vi "test-CSM mode.vi"(8 "error in (no error)":errorcluster, 11 "TestCase in":refnum<class "testcase-CSMAttributes.lvclass">) -> (0 "error out":errorcluster, 3 "TestCase out":refnum<class "testcase-CSMAttributes.lvclass">)   [LabVIEW 2017, in "testcase-CSMAttributes.lvclass"]
uses:
  testcase-CSMAttributes.lvclass
  5e1fa0b9-9953-4aea-b14f-852d0926f464.vi
  ca6da20f-918c-4697-94f5-fe779df5fb56.vi
  b6cafa74-5be5-493d-85c2-392da22f0834.vi
  474ebc5b-ede4-4fe2-a33b-3b2c34e901f1.vi
  6dc37769-ead1-45fc-a673-d21298543349.vi
  2b38d03e-680a-4e35-9447-0bd23ed7c194.vi
  aa53e100-d513-4525-b5da-2cac676b671d.vi
  src/user.lib/_NEVSTOP/Communicable State Machine(CSM)/AdvanceAPI/CSM - Set Module Attribute.vi
  src/user.lib/_NEVSTOP/Communicable State Machine(CSM)/AdvanceAPI/CSM - Get Module Attribute.vi
  <vilib>/addons/_JKI Toolkits/VI Tester/TestCase.llb/TestCase.lvclass
  src/user.lib/_NEVSTOP/Communicable State Machine(CSM)/Communicable State Machine.lvlib
  C:/Program Files (x86)/National Instruments/LabVIEW 2017/vi.lib/addons/_JKI Toolkits/VI Tester/TestCase.llb/TestCase.lvclass
panel:
  out "error out":errorcluster
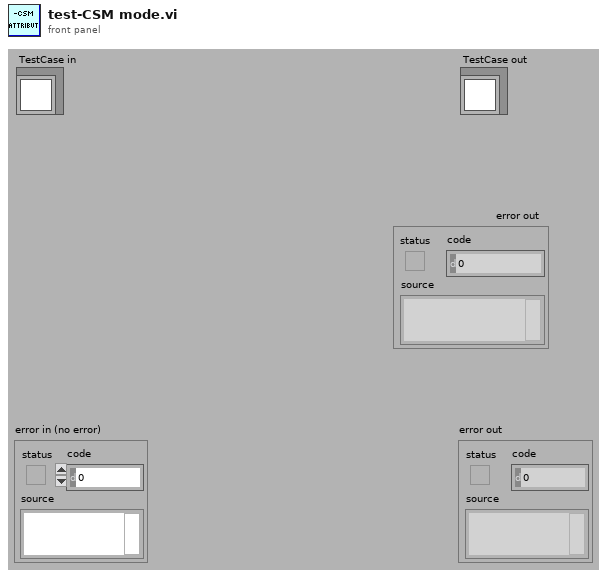
[diagram p1: front panel]
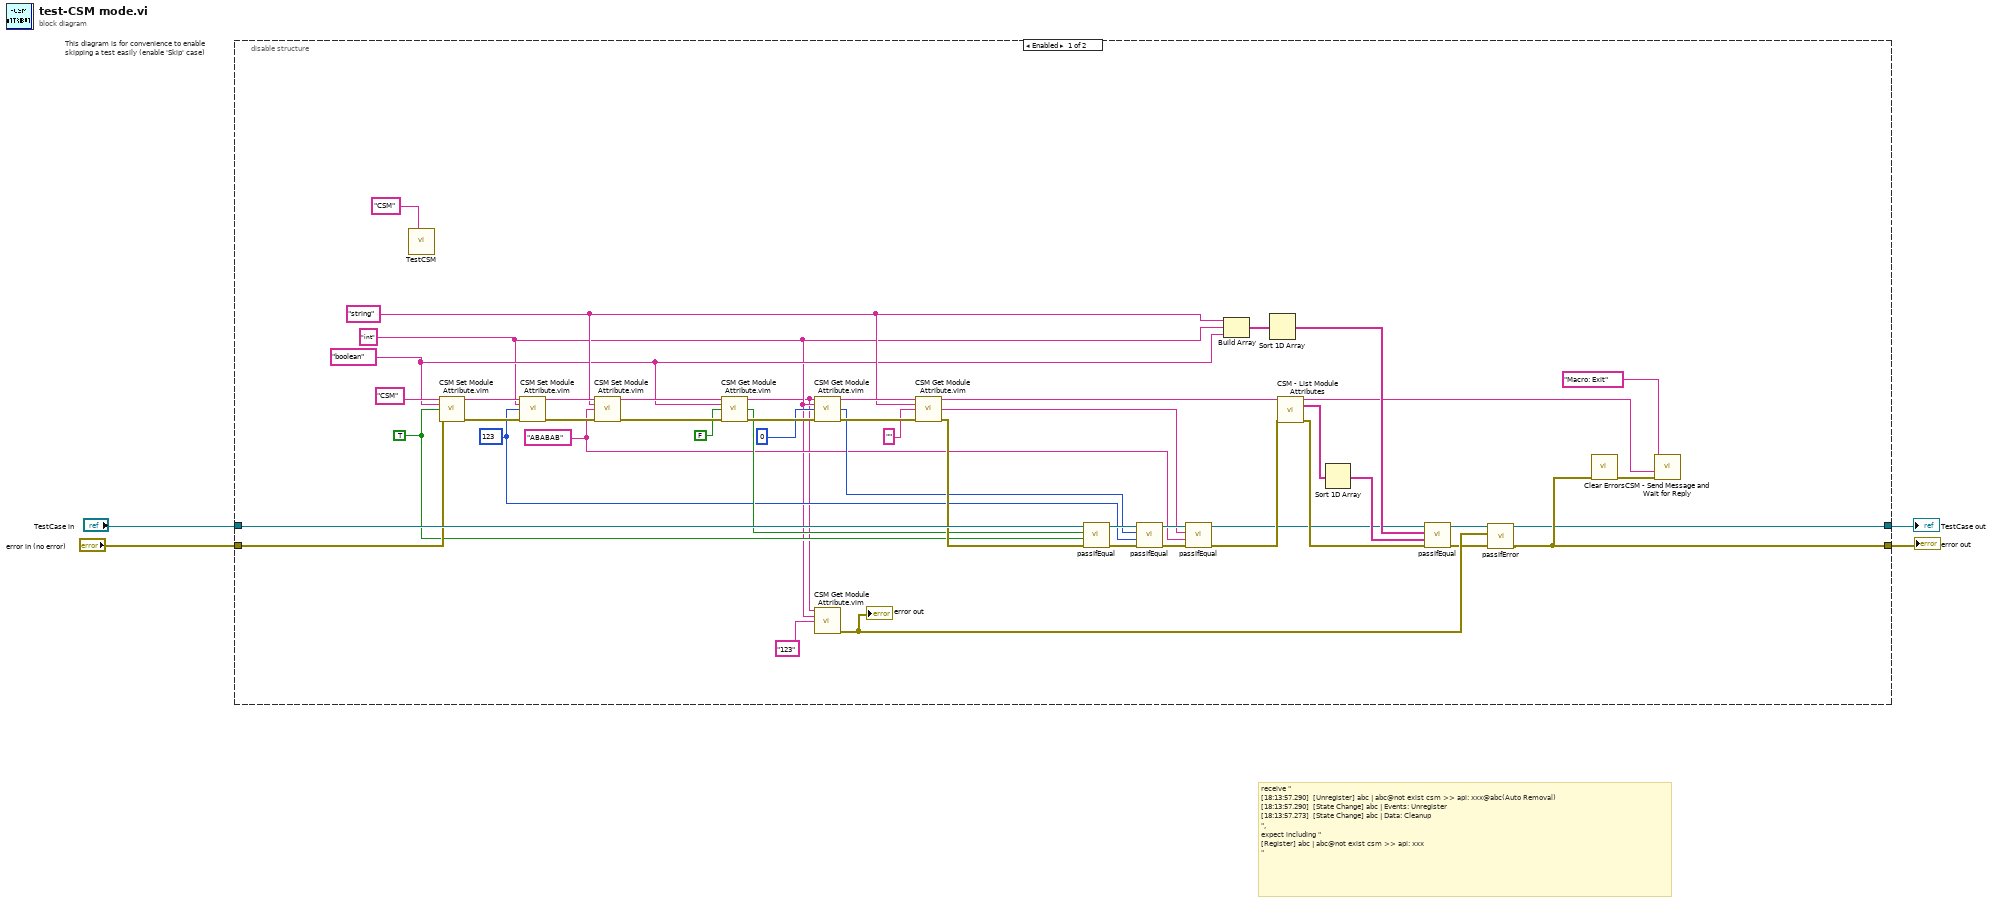
[diagram p0: block diagram]
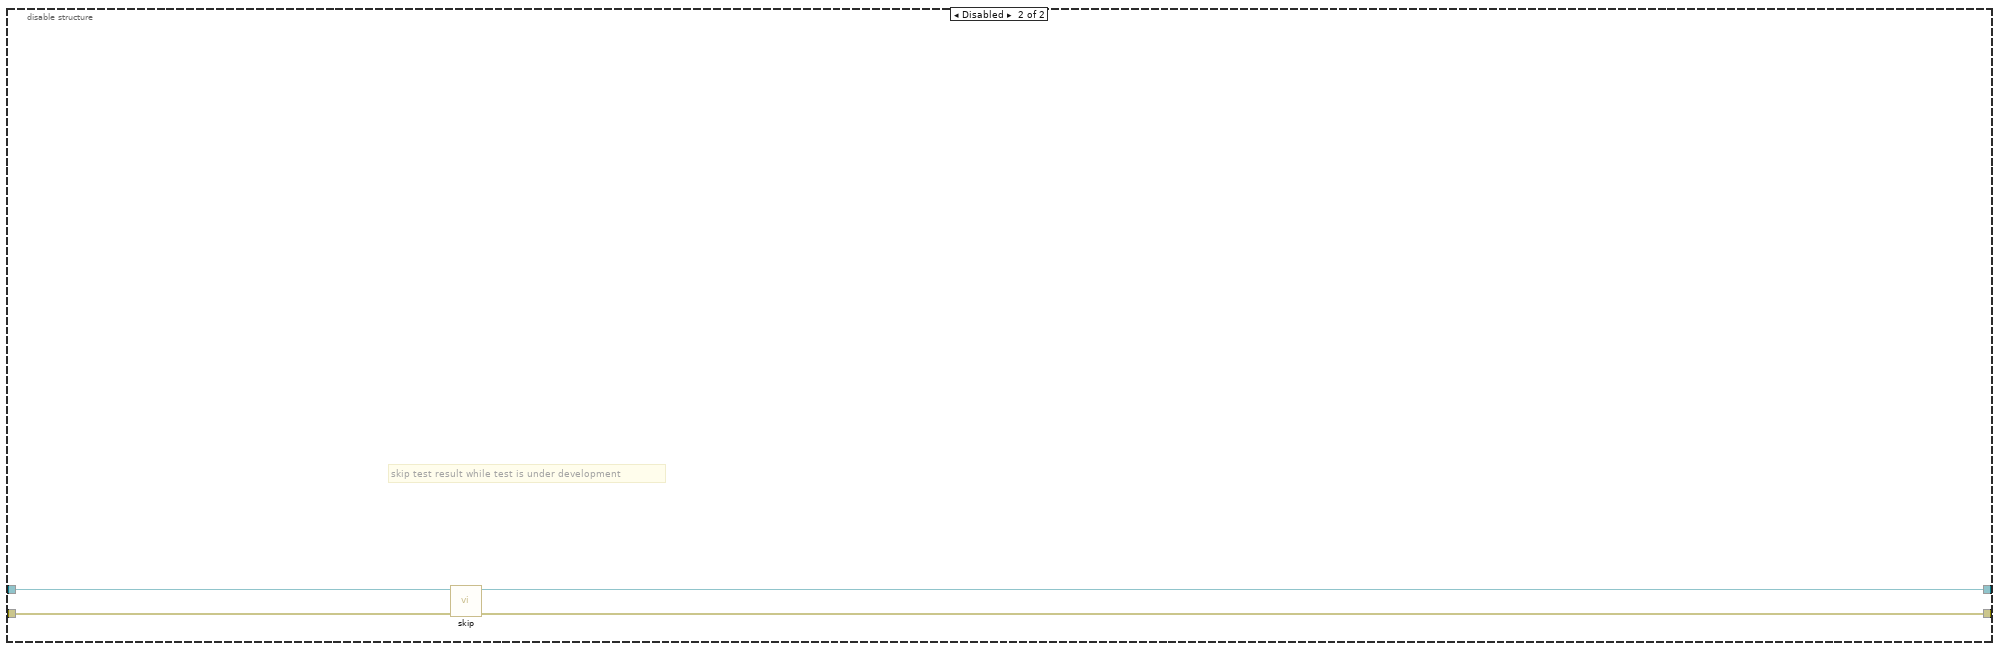
[diagram p2: hidden frame]
diagram:
  # "receive \"\n[18:13:57.290]  [Unregister] abc | abc@not exist csm >> api: xxx@abc(Auto Removal)\n[18:13:57.290]  [State Change] abc | Events: Unregister\n[18:13:57.273]  [State Change] abc | Data: Cleanup\n\", \nexpect including \"\n[Register] abc | abc@not exist csm >> api: xxx\n\""
  n1 = disable-structure "This diagram is for convenience to enable skipping a test easily (enable 'Skip' case)" shown="Enabled" {
    disable-tunnel: "TestCase in" -> [w52 w56]
    disable-tunnel: [w5 w54] -> w1
    disable-tunnel: [w6 w55] -> w3
    disable-tunnel: "error in (no error)" -> [w51 w53]
    frame Enabled {
      w26 = "ABABAB" ("Attribute")
      w22 = "string" ("Attribute")
      w30 = 123
      w11 = "int" ("Attribute")
      w35 = TRUE
      w21 = "boolean" ("Attribute")
      n2 = call "TestCSM.vi"("Name (\"\" to Use UUID)"="CSM" ("Name (\"\" to Use UUID)")) -> ()  [unwired: 11 in]
      n3 = call "CSM Set Module Attribute.vim"("CSM Name"="CSM" ("Name (\"\" to Use UUID)"), "Attribute"=w21, "Value"=w35, "Error In"=w51) -> ("CSM Name (Dup)"=w46:string, "error out"=w48:errorcluster)  [unwired: 8 in, 2 out]
      n4 = call "CSM Set Module Attribute.vim"("CSM Name"=w46, "Attribute"=w11, "Value"=w30, "Error In"=w48) -> ("CSM Name (Dup)"=w45:string, "error out"=w47:errorcluster)  [unwired: 8 in, 2 out]
      n5 = call "CSM Set Module Attribute.vim"("CSM Name"=w45, "Attribute"=w22, "Value"=w26, "Error In"=w47) -> ("CSM Name (Dup)"=w43:string, "error out"=w44:errorcluster)  [unwired: 8 in, 2 out]
      n6 = call "CSM Get Module Attribute.vim"("CSM Name"=w43, "Attribute"=w21, "Default Value (Empty Variant)"=FALSE, "Error In"=w44) -> ("CSM Name (Dup)"=w10:string, "Value"=w34:bool, "error out"=w42:errorcluster)  [unwired: 7 in, 2 out]
      n7 = call "CSM Get Module Attribute.vim"("CSM Name"=w10, "Attribute"=w11, "Default Value (Empty Variant)"=0, "Error In"=w42) -> ("CSM Name (Dup)"=w41:string, "Value"=w31:i32, "error out"=w40:errorcluster)  [unwired: 7 in, 2 out]
      n8 = call "CSM Get Module Attribute.vim"("CSM Name"=w10, "Attribute"=w11, "Default Value (Empty Variant)"="123") -> ("error out"=w8:errorcluster)  [unwired: 8 in, 4 out]
      "error out" <- w8
      n9 = call "CSM Get Module Attribute.vim"("CSM Name"=w41, "Attribute"=w22, "Default Value (Empty Variant)"="" ("Attribute"), "Error In"=w40) -> ("CSM Name (Dup)"=w25:string, "Value"=w27:string, "error out"=w36:errorcluster)  [unwired: 7 in, 2 out]
      n10 = call-dynamic "passIfEqual.vi"("error in (no error)"=w36, "y"=w35, "x"=w34, "TestCase in"=w52) -> ("error out"=w32:errorcluster, "TestCase out"=w33:refnum<class "testcase-CSMAttributes.lvclass">)  [unwired: 6 in]
      n11 = call-dynamic "passIfEqual.vi"("error in (no error)"=w32, "y"=w30, "x"=w31, "TestCase in"=w33) -> ("error out"=w28:errorcluster, "TestCase out"=w29:refnum<class "testcase-CSMAttributes.lvclass">)  [unwired: 6 in]
      n12 = call-dynamic "passIfEqual.vi"("error in (no error)"=w28, "y"=w26, "x"=w27, "TestCase in"=w29) -> ("error out"=w24:errorcluster, "TestCase out"=w16:refnum<class "testcase-CSMAttributes.lvclass">)  [unwired: 6 in]
      n13 = Build Array(w22, w11, w21) -> (w20:string[])
      n14 = Sort 1D Array(array=w20) -> (sorted array=w17:string[])
      n15 = call "CSM - List Module Attributes.vi"("CSM Name"=w25, "Error In"=w24) -> ("CSM Name (Dup)"=w14:string, "Attributes"=w19:string[], "error out"=w23:errorcluster)  [unwired: 9 in, 2 out]
      n16 = Sort 1D Array(array=w19) -> (sorted array=w18:string[])
      n17 = call-dynamic "passIfEqual.vi"("error in (no error)"=w23, "y"=w18, "x"=w17, "TestCase in"=w16) -> ("error out"=w7:errorcluster, "TestCase out"=w9:refnum<class "testcase-CSMAttributes.lvclass">)  [unwired: 6 in]
      n18 = call-dynamic "passIfError.vi"("error in (no error)"=w7, "error"=w8, "TestCase in"=w9) -> ("error out"=w6:errorcluster, "TestCase out"=w5:refnum<class "testcase-CSMAttributes.lvclass">)  [unwired: 7 in]
      n19 = call <vilib>:"Clear Errors.vi"("error in (no error)"=w6) -> ("error out"=w15:errorcluster)  [unwired: 5 in, 1 out]
      n20 = call "CSM - Send Message and Wait for Reply.vi"("Error In (No Error)"=w15, "Target Module"=w14, "State"="Macro: Exit") -> ()  [unwired: 6 in, 3 out]
    }
    frame Disabled {
      # "skip test result while test is under development"
      n21 = call <vilib>:"skip.vi"("error in (no error)"=w53, "TestCase in"=w56) -> ("error out"=w55:errorcluster, "TestCase out"=w54:refnum<class "testcase-CSMAttributes.lvclass">)  [unwired: 8 in]
    }
  }
  "error out" <- w3
  "TestCase out" <- w1
